vi "Cron Basic Scheduler Template.vi"   [LabVIEW 2013]
uses:
  Cron/Create Cron Job.vi
  Cron/Compute Next Cron.vi
  Cron.Quartz/Cron.Quartz.lvclass
  openCron.lvlib
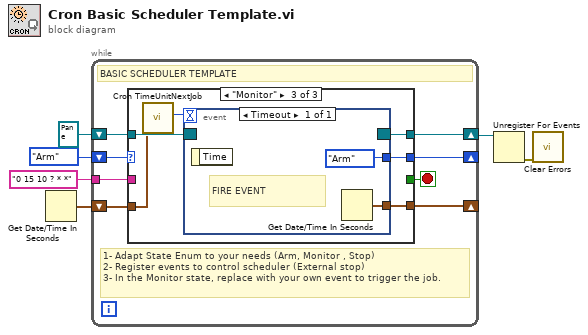
[diagram p0: block diagram]
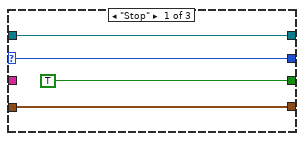
[diagram p2: hidden frame]
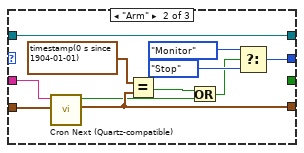
[diagram p3: hidden frame]
diagram:
  n1 = Get Date/Time In Seconds() -> (seconds since 1Jan1904=w6:timestamp)
  n2 = while {
    shift-right: [w13] -> _
    shift-left: w6 -> [w14]
    tunnel: "0 15 10 ? * *" -> [w12]
    shift-right: [w10] -> _
    shift-left: enum16{"Arm", "Stop", "Monitor"}."Arm" -> [w11]
    shift-right: [w7] -> w2
    shift-left: refnum<event-registration> refnum ("event registration refnum") -> [w8]
    stop <- w9 stop-if-true
    # "1- Adapt State Enum to your needs (Arm, Monitor , Stop)\n2- Register events to control scheduler (External stop)\n3- In the Monitor state, replace with your own event to trigger the job."
    # "BASIC SCHEDULER TEMPLATE"
    n3 = case shown="\"Monitor\"" w11 {
      selector: w11 -> [w18 _ _]
      tunnel: w14 -> [w16 w29 w30]
      tunnel: [w16 w23 w32] -> w13
      tunnel: w12 -> [_ w28 _]
      tunnel: [w18 w26 w33] -> w10
      tunnel: [TRUE _ _] -> w9
      tunnel: w8 -> [w15 w24 w35]
      tunnel: [w15 w24 w34] -> w7
      frame "Stop" {
      }
      frame "Arm" {
        n4 = call "Cron Next (Quartz-compatible).vi"("Reference timestamp (Now)"=w29, "Cron Expression"=w28) -> ("Next Occurence"=w23:timestamp, "syntax valid?"=w20:bool)  [unwired: 7 in, 1 out]
        n5 = Equal?(x=timestamp(0 s since 1904-01-01) ("y"), y=w23) -> (x = y?=w21:bool)
        n6 = Or(x=w21, y=w20) -> (x .or. y?=w19:bool)
        n7 = Select(t=enum16{"Arm", "Stop", "Monitor"}."Monitor", s=w19, f=enum16{"Arm", "Stop", "Monitor"}."Stop") -> (s? t:f=w26:enum16{"Arm", "Stop", "Monitor"})
      }
      frame "Monitor" {
        n8 = call "Cron TimeUnitNextJob.vi"("Next Occurence"=w30) -> ("next event (ms)"=w31:i32)  [unwired: 10 in]
        n9 = event shown="[0] Timeout" {
          selector: w35 -> [_]
          dyn-events: [_] -> w34
          timeout: w31 -> [_]
          tunnel: [enum16{"Arm", "Stop", "Monitor"}."Arm"] -> w33
          tunnel: [w36] -> w32
          event Timeout {
            # "FIRE EVENT"
            n10 = event-data() -> ()  [unwired: 1 in, 1 out]
            n11 = Get Date/Time In Seconds() -> (seconds since 1Jan1904=w36:timestamp)
          }
        }
      }
    }
  }
  n12 = Unregister For Events(event registration refnum=w2) -> (error out=w1:errorcluster)  [unwired: 1 in]
  n13 = call <vilib>:"Clear Errors.vi"("error in (no error)"=w1) -> ()  [unwired: 6 in, 1 out]
